vi "Process.vi"(8 "error in (no error)":errorcluster, 10 "Pound in":refnum<class "Pound.lvclass">, 11 "Qbus in":refnum<class "Qbus.lvclass">) -> (0 "error out":errorcluster)   [LabVIEW 2017, in "Loop7.lvlib"]
uses:
  <vilib>/addons/InsightCM/Devices/Shared/Common/DataFlow/test/SpeedBenchmark/Loop7/Loop7.lvlib
  <vilib>/addons/InsightCM/Devices/Shared/Common/DataFlow/test/SpeedBenchmark/Loop7/controls/state.ctl
  <vilib>/addons/Qbus/Qbus.lvclass
  <vilib>/addons/InsightCM/Devices/Shared/Common/DataFlow/test/SpeedBenchmark/Loop7/controls/config.ctl
  <vilib>/addons/Qbus/controls/state.ctl
  <vilib>/NI/Software Watchdog/Watchdog/Watchdog.lvclass
  <vilib>/addons/InsightCM/Devices/Shared/Common/DataFlow/DataFlow.lvlib
  <vilib>/NI/Software Watchdog/Pound/Pound.lvclass
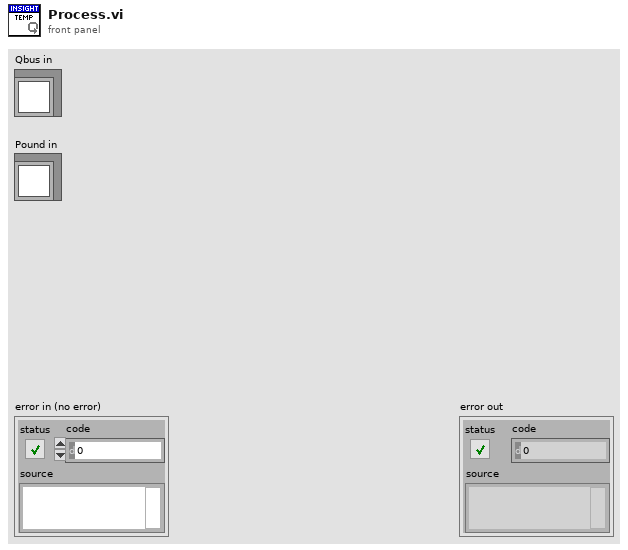
[diagram p1: front panel]
types:
  T1 = typedef "Loop7.lvlib/config.ctl" = cluster{"placeholder":string}
  T2 = typedef "Loop7.lvlib/state.ctl" = enum16{"Idle", "Ready", "Live"}
  T3 = typedef "Qbus.lvclass/state.ctl" = enum16{"unconfigured", "configured"}
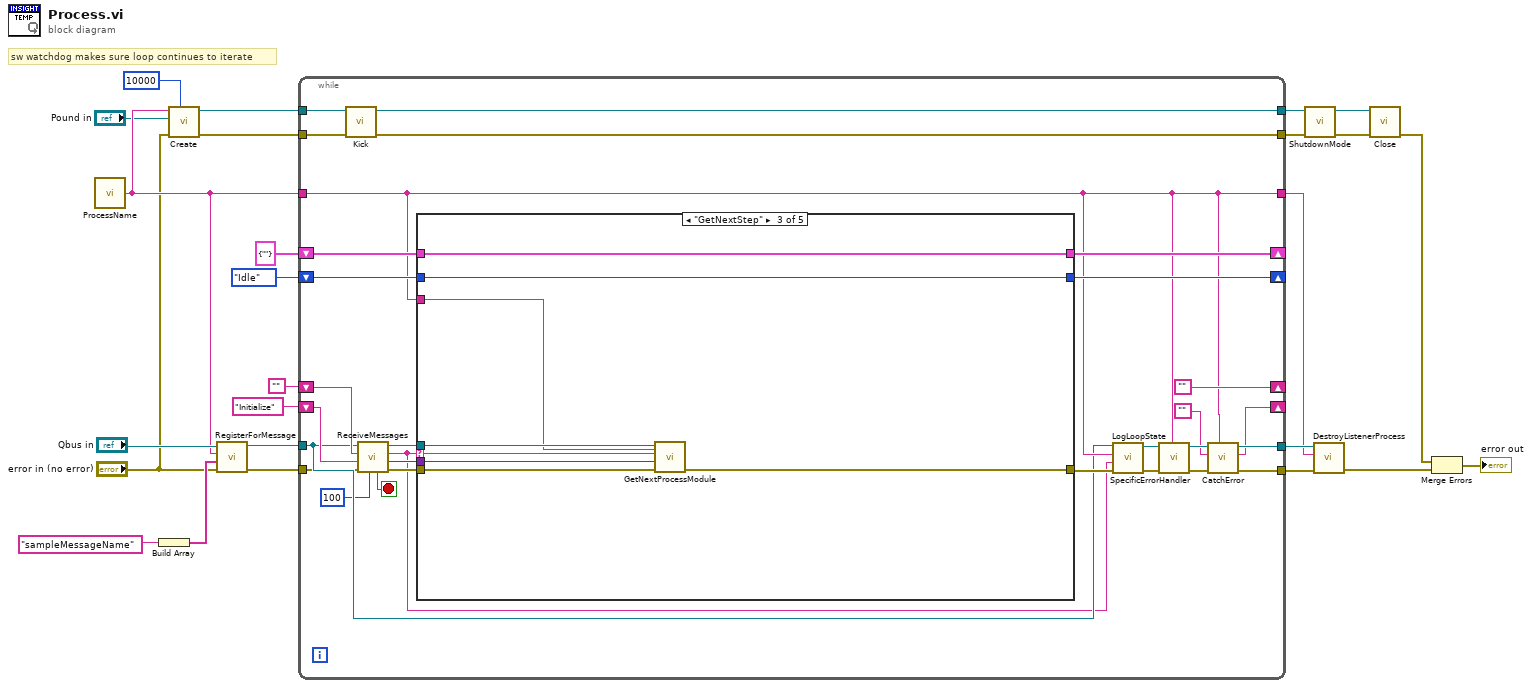
[diagram p0: block diagram]
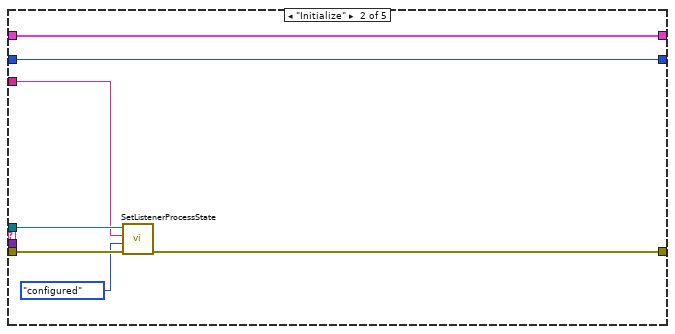
[diagram p3: hidden frame]
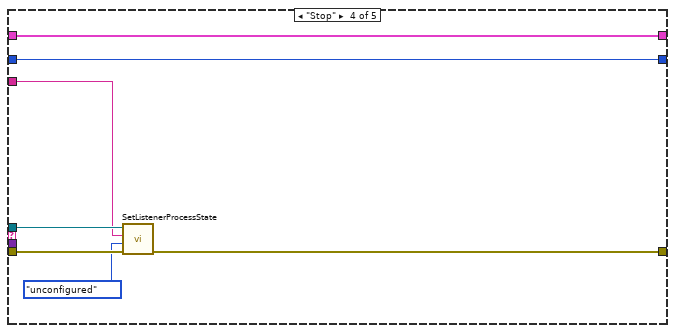
[diagram p4: hidden frame]
diagram:
  # "sw watchdog makes sure loop continues to iterate"
  n1 = call <vilib>:"ProcessName.vi"() -> ("ProcessName"=w13:string)  [unwired: 5 in]
  n2 = Build Array("sampleMessageName" ("String")) -> (w14:string[])
  n3 = call <vilib>:"Create.vi"("Execution Timeout (ms)"=u32 10000, "error in (no error)"="error in (no error)", "Pound"="Pound in", "Name"=w13) -> ("error out"=w6:errorcluster, "Watchdog"=w12:refnum<data-value>)  [unwired: 6 in]
  n4 = call <vilib>:"RegisterForMessage.vi"("error in (no error)"="error in (no error)", "message names"=w14, "process name"=w13, "Qbus in"="Qbus in") -> ("error in (no error)"=w23:errorcluster, "Qbus out"=w22:refnum<class "Qbus.lvclass">)  [unwired: 6 in]
  n5 = while {
    tunnel: w23 -> [w29]
    shift-right: [w50] -> _
    shift-left: state."Idle" ("state") -> [w53]
    shift-right: [""] -> _
    shift-left: "" -> [w52]
    tunnel: [w42] -> w21
    tunnel: w22 -> [w34]
    tunnel: w13 -> [w35]
    tunnel: [w40] -> w20
    tunnel: [w35] -> w19
    shift-right: [w38] -> _
    shift-left: "Initialize" -> [w46]
    shift-right: [w44] -> _
    shift-left: T1 {"placeholder"=""} ("config") -> [w45]
    tunnel: w12 -> [w32]
    tunnel: [w31] -> w8
    tunnel: w6 -> [w30]
    tunnel: [w28] -> w5
    stop <- w54 stop-if-true
    n6 = call <vilib>:"Kick.vi"("error in (no error)"=w30, "Watchdog"=w32) -> ("error out"=w28:errorcluster, "Watchdog"=w31:refnum<data-value>)  [unwired: 8 in]
    n7 = call <vilib>:"ReceiveMessages.vi"("Timeout(100)"=100 ("milliseconds to wait"), "error in (no error)"=w29, "Priority Action"=w46, "Default Action"=w52, "Qbus in"=w34) -> ("error out"=w51:errorcluster, "MsgValue"=w47:variant, "Action"=w27:string, "Qbus out"=w48:refnum<class "Qbus.lvclass">, "Exit"=w54:bool)  [unwired: 2 in]
    n8 = case shown="\"GetNextStep\"" w27 {
      selector: w27 -> [_ _ w66 _ _]
      tunnel: w53 -> [w57 w64 w72 w79 w82]
      tunnel: w51 -> [w56 w62 w70 w77 w81]
      tunnel: w48 -> [_ w61 w68 w75 _]
      tunnel: [w56 w60 w69 w76 w81] -> w37
      tunnel: [w57 w64 w72 w79 w82] -> w50
      tunnel: w47 -> [_ _ w67 _ _]
      tunnel: w45 -> [w55 w63 w71 w78 w80]
      tunnel: [w55 w63 w71 w78 w80] -> w44
      tunnel: w35 -> [_ w59 w65 w74 _]
      frame "", Default {
      }
      frame "Initialize" {
        n9 = call <vilib>:"SetListenerProcessState.vi"("error in (no error)"=w62, "state"=state."configured", "ProcessName"=w59, "Qbus in"=w61) -> ("error out"=w60:errorcluster)  [unwired: 6 in, 1 out]
      }
      frame "GetNextStep" {
        n10 = call <vilib>:"GetNextProcessModule.vi"(7:w65, "error in (no error)"=w70, "data"=w67, "source"=w66, "Qbus in"=w68) -> ("error out"=w69:errorcluster)  [unwired: 5 in, 1 out]
      }
      frame "Stop" {
        n11 = call <vilib>:"SetListenerProcessState.vi"("error in (no error)"=w77, "state"=state."unconfigured", "ProcessName"=w74, "Qbus in"=w75) -> ("error out"=w76:errorcluster)  [unwired: 6 in, 1 out]
      }
      frame "Exit" {
      }
    }
    n12 = call <vilib>:"LogLoopState.vi"("error in (no error)"=w37, "loop action"=w27, "process name"=w35, "Qbus in"=w34) -> ("error out"=w36:errorcluster, "Qbus out"=w33:refnum<class "Qbus.lvclass">)  [unwired: 6 in]
    n13 = call <vilib>:"SpecificErrorHandler.vi"("error in (no error)"=w36, "ProcessName"=w35, "Qbus in"=w33) -> ("error out"=w43:errorcluster, "Qbus out"=w41:refnum<class "Qbus.lvclass">)  [unwired: 7 in]
    n14 = call <vilib>:"CatchError.vi"("source"=w35, "error in (no error)"=w43, "next action in"="", "Qbus in"=w41) -> ("error out"=w42:errorcluster, "next action out"=w38:string, "Qbus out"=w40:refnum<class "Qbus.lvclass">)  [unwired: 5 in]
  }
  n15 = call <vilib>:"ShutdownMode.vi"("error in (no error)"=w5, "Watchdog"=w8) -> ("error out"=w7:errorcluster, "Watchdog"=w9:refnum<data-value>)  [unwired: 8 in]
  n16 = call <vilib>:"DestroyListenerProcess.vi"("error in (no error)"=w21, "process name"=w19, "Qbus in"=w20) -> ("error in (no error)"=w4:errorcluster)  [unwired: 7 in, 1 out]
  n17 = call <vilib>:"Close.vi"("error in (no error)"=w7, "Watchdog"=w9) -> ("error out"=w3:errorcluster)  [unwired: 9 in]
  n18 = Merge Errors(w3, w4) -> (→"error out":errorcluster)
